vi "Simple Encoder Test GUI.vi"() -> ()   [LabVIEW 2009]
uses:
  Strict Raw Encoder Cluster.ctl
  <vilib>/userDefined/High Color/nirio_resource_hc.ctl
  <vilib>/rvi/interface/nirviOpenFPGA/nirviOpenFPGA.xnode
  FPGA Bitfiles/Athena Brain.lvproj_FPGA Target 2_SuperSimpleEncoder~0F.lvbitx
  <vilib>/FPGAPlugInAG/sbRIO-9642/nirviIntfOpen_sbRIO-9642.vi
  <vilib>/rvi/interface/nirviReadWriteControl/nirviReadWriteControl.xnode
  <vilib>/Utility/error.llb/Error Cluster From Error Code.vi
  <vilib>/rvi/errors/niLvFpgaAdjustHostInterfaceError.vi
  <vilib>/rvi/interface/common/niFpgaNodeNameForErrorReporting.ctl
  <vilib>/rvi/errors/niLvFpgaWhatHappensToTopLevelVI.ctl
  <vilib>/rvi/interface/nirviCloseFPGA/nirviCloseFPGA.xnode
  <vilib>/FPGAPlugInAG/sbRIO-9642/nirviIntfClose_sbRIO-9642.vi
  NiRioSrv.dll
panel:
  out "Count Zeroed at Index":i32
  out "Count Zeroed at Fake Index":i32
  out "Current  Fake count":i32
  out "Port2/DIO0":bool
  in  "Use Port2/DIO0 to control Fake Lidar Encoder Index":bool
  in  "Fake Lidar Encoder Index":bool
  in  "Index Point":i32=2000
  in  "Reader Stop":bool
  out "Steering Encoder":i32
  out "Lidar Encoder":i32
  out "Drive Encoder":i32
  out "Encoder Information":T1
  in  "stop":bool
  in  "Lidar Enable":bool
  in  "Steering Enable":bool
  in  "Drive Enable":bool
  in  "Lidar output Voltage":fxp<+/-,20,5> format="%.17g"
  in  "Steering output Voltage":fxp<+/-,20,5> format="%.17g"
  in  "Drive output Voltage":fxp<+/-,20,5> format="%.17g"
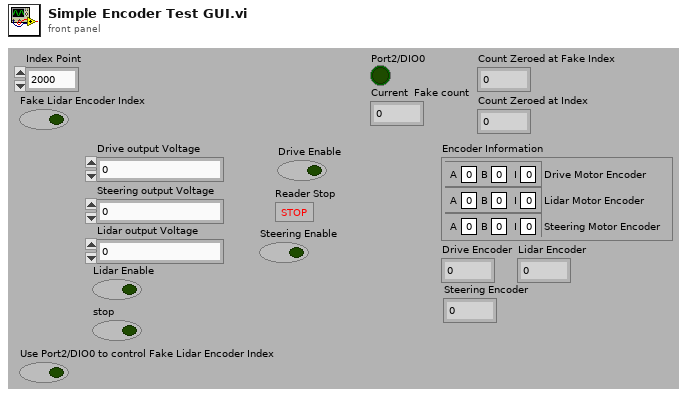
[diagram p1: front panel]
types:
  T1 = typedef "Strict Raw Encoder Cluster.ctl" = cluster{"Drive Motor Encoder":cluster{"A":bool, "B":bool, "I":bool}, "Lidar Motor Encoder":cluster{"A":bool, "B":bool, "I":bool}, "Steering Motor Encoder":cluster{"A":bool, "B":bool, "I":bool}}
  T2 = typedef "nirio_resource_hc.ctl" = tag
  T3 = typedef "niFpgaNodeNameForErrorReporting.ctl" = enum16{"Open FPGA VI Reference", "Read/Write Control", "Invoke Method: Abort", "Invoke Method: Acknowledge IRQ", "Invoke Method: Download", "Invoke Method: FIFO.Configure", "Invoke Method: FIFO.Read", "Invoke Method: FIFO.Start", "Invoke Method: FIFO.Stop", "Invoke Method: FIFO.Write", "Invoke Method: Reset", "Invoke Method: Run", "Invoke Method: Wait on IRQ", "Close FPGA VI Reference"}
  T4 = typedef "niLvFpgaWhatHappensToTopLevelVI.ctl" = enum16{"top level VI scripted behind XNode", "top level VI inlined behind XNode"}
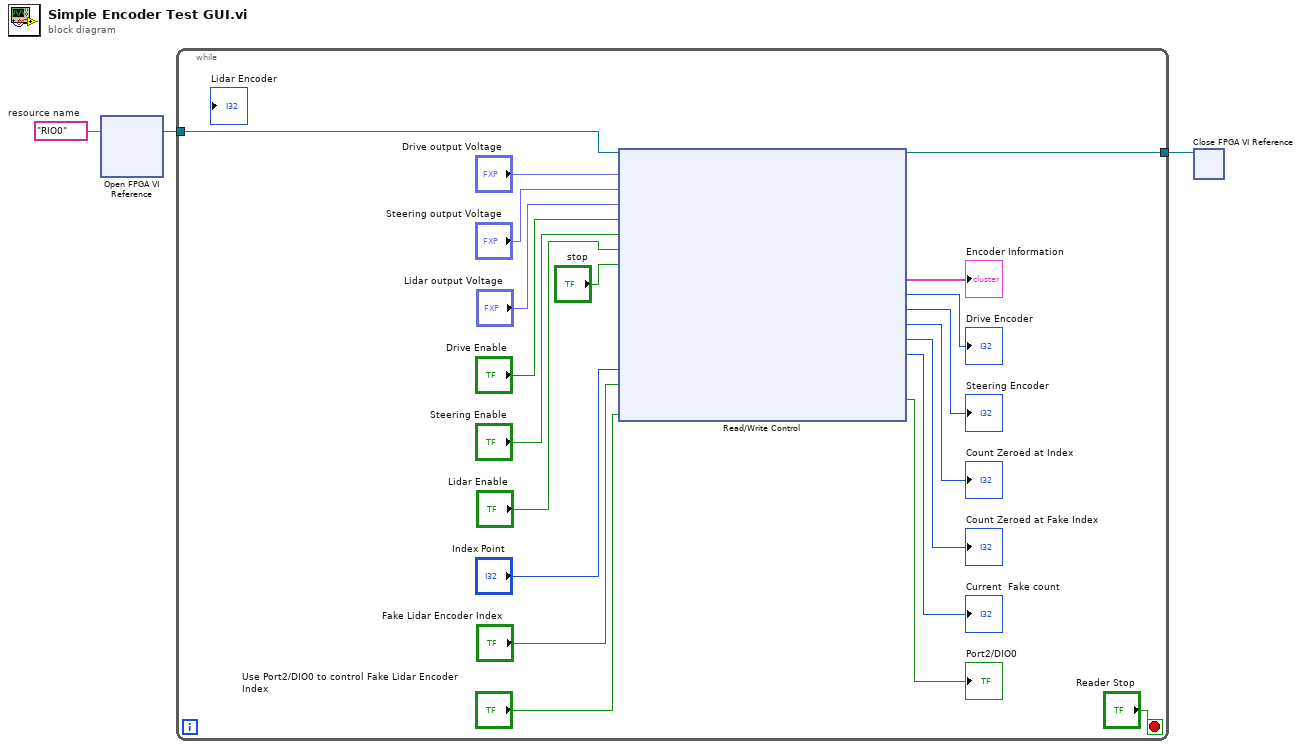
[diagram p0: block diagram]
diagram:
  w2 = T2 "RIO0"  # resource name
  n1 = xnode "Open FPGA VI Reference"("resource name"=w2) -> ("FPGA VI Reference Out"=w3:refnum<k20>)  [unwired: 1 in, 1 out]
  n2 = while {
    tunnel: w3 -> [w23]
    tunnel: [w12] -> w1
    stop <- "Reader Stop" stop-if-true
    n3 = xnode "Read/Write Control"("FPGA VI Reference In"=w23, "Drive output Voltage"="Drive output Voltage", "Steering output Voltage"="Steering output Voltage", "Lidar output Voltage"="Lidar output Voltage", "Drive Enable"="Drive Enable", "Steering Enable"="Steering Enable", "Lidar Enable"="Lidar Enable", "stop"="stop", "Index Point"="Index Point", "Fake Lidar Encoder Index"="Fake Lidar Encoder Index", "Use Port2/DIO0 to control Fake Lidar Encoder Index"="Use Port2/DIO0 to control Fake Lidar Encoder Index") -> ("FPGA VI Reference Out"=w12:refnum<k20>, "Encoder Information"=→"Encoder Information":T1, "Drive Encoder"=→"Drive Encoder":i32, "Steering Encoder"=→"Steering Encoder":i32, "Count Zeroed at Index"=→"Count Zeroed at Index":i32, "Count Zeroed at Fake Index"=→"Count Zeroed at Fake Index":i32, "Current  Fake count"=→"Current  Fake count":i32, "Port2/DIO0"=→"Port2/DIO0":bool)  [unwired: 1 in, 1 out]
  }
  n4 = xnode "Close FPGA VI Reference"("FPGA VI Reference In"=w1) -> ()  [unwired: 1 in, 1 out]
